vi "GetType.vi"(8 "error in (no error)":errorcluster, 11 "Add Value without TS Msg":refnum<class "Add Value without TS Msg.lvclass">) -> (0 "error out":errorcluster, 2 "Data Sample":variant, 3 "Add Value without TS Msg":refnum<class "Add Value without TS Msg.lvclass">)   [LabVIEW 2019, in "BNT_XtGraph.lvlib" / "Add Value without TS Msg.lvclass"]
uses:
  Add Value without TS Msg.lvclass
  Add Value without TS Msg.lvclass/Add Value without TS Msg.ctl
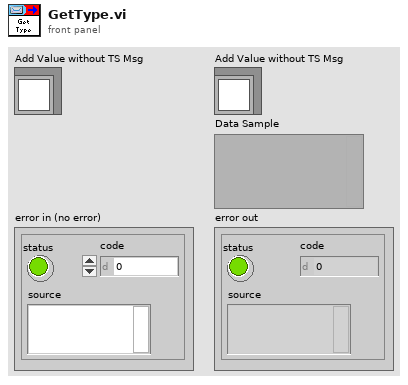
[diagram p1: front panel]
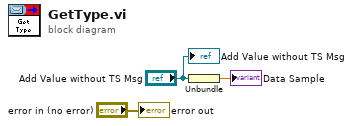
[diagram p0: block diagram]
diagram:
  n1 = Unbundle("Add Value without TS Msg") -> (→"Data Sample":dbl)
  "error out" <- "error in (no error)"
  "Add Value without TS Msg" <- "Add Value without TS Msg"
